vi "Gunsim Initial Position.vi"(1 "Parameters":T1, 2 "Robot Constants":T3={"Distance from Pivot Point to Drive Mount(in)"=2.0, "Distance from Pivot Point to Arm Mount(in)"=2.0, "Distance from Pivot Point to Launcher(in)"=2.0, "Distance from Pivot Point to Camera(in)"=2.0, "WheelEncoder Ticks/Revolution"=2.0, "Wheel Radius"=2.0, "Triangle Angle(degrees)"=2.0, "Minimum LA Distance(inches)"=2.0, "LA Distance/Tick(inches)"=2.0}, 3 "cluster in":T2) -> (0 "cluster out":T2)   [LabVIEW 2015]
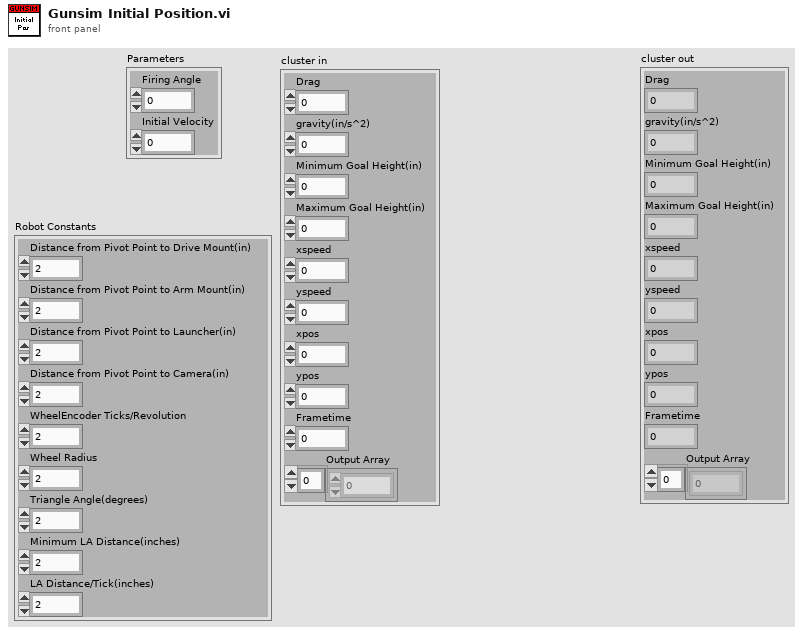
[diagram p1: front panel]
types:
  T1 = cluster{"Firing Angle":dbl, "Initial Velocity":dbl}
  T2 = cluster{"Drag":dbl, "gravity(in/s^2)":dbl, "Minimum Goal Height(in)":dbl, "Maximum Goal Height(in)":dbl, "xspeed":dbl, "yspeed":dbl, "xpos":dbl, "ypos":dbl, "Frametime":dbl, "Output Array":dbl[]}
  T3 = cluster{"Distance from Pivot Point to Drive Mount(in)":dbl, "Distance from Pivot Point to Arm Mount(in)":dbl, "Distance from Pivot Point to Launcher(in)":dbl, "Distance from Pivot Point to Camera(in)":dbl, "WheelEncoder Ticks/Revolution":dbl, "Wheel Radius":dbl, "Triangle Angle(degrees)":dbl, "Minimum LA Distance(inches)":dbl, "LA Distance/Tick(inches)":dbl}
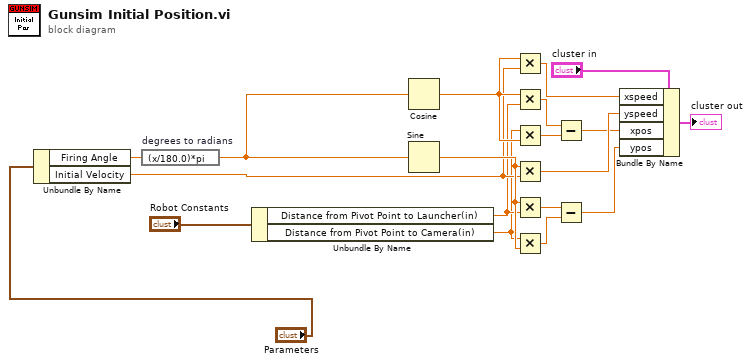
[diagram p0: block diagram]
diagram:
  n1 = Unbundle By Name("Parameters") -> ("Firing Angle"=w17:dbl, "Initial Velocity"=w7:dbl)
  n2 = expression code="(x/180.0)*pi" "degrees to radians"(w17) -> (w16:dbl)
  n3 = Unbundle By Name("Robot Constants") -> ("Distance from Pivot Point to Launcher(in)"=w6:dbl, "Distance from Pivot Point to Camera(in)"=w5:dbl)
  n4 = Cosine(x=w16) -> (cos(x)=w13:dbl)
  n5 = Sine(x=w16) -> (sin(x)=w11:dbl)
  n6 = Multiply(x=w13, y=w7) -> (x*y=w19:dbl)
  n7 = Multiply(x=w13, y=w6) -> (x*y=w14:dbl)
  n8 = Multiply(x=w5, y=w13) -> (x*y=w12:dbl)
  n9 = Multiply(x=w11, y=w7) -> (x*y=w18:dbl)
  n10 = Multiply(x=w11, y=w6) -> (x*y=w15:dbl)
  n11 = Multiply(x=w5, y=w11) -> (x*y=w10:dbl)
  n12 = Subtract(x=w14, y=w12) -> (x-y=w8:dbl)
  n13 = Subtract(x=w15, y=w10) -> (x-y=w9:dbl)
  n14 = Bundle By Name(cluster="cluster in", "xspeed"=w19, "yspeed"=w18, "xpos"=w8, "ypos"=w9) -> (→"cluster out":T2)
